vi "Stop Work.vi"(6 "Controller name":string, 8 "error in (no error)":errorcluster, 9 "Reply":bool=TRUE, 10 "Reply to":refnum<class "Stop Response Msg.lvclass">, 11 "Measure Object in":refnum<class "Channel Scanner.lvclass">) -> (0 "error out":errorcluster, 3 "Measure Object out":refnum<class "Channel Scanner.lvclass">)   [LabVIEW 2021, in "Channel Scanner.lvclass"]
uses:
  Channel Scanner.lvclass
  C:/Program Files/National Instruments/LabVIEW 2021/vi.lib/ActorFramework/Actor/Actor.lvclass
  Controllers/Process Controller Messages/Stop Response Msg/Stop Response Msg.lvclass
  <vilib>/ActorFramework/Actor/Actor.lvclass/Actor.ctl
  <vilib>/ActorFramework/Message Enqueuer/Message Enqueuer.lvclass/Message Enqueuer.ctl
  Publish-Subscribe/Interfaces/Publisher Messages/Unsubscribe Msg/Unsubscribe Msg.lvclass/Unsubscribe Msg.ctl
  <vilib>/ActorFramework/Message Enqueuer/Init from Existing Queue.vi
  <vilib>/ActorFramework/Message Enqueuer/Enqueue.vi
  Publish-Subscribe/Interfaces/Publisher Messages/Unsubscribe Msg/Unsubscribe Msg.lvclass
  C:/Program Files/National Instruments/LabVIEW 2021/vi.lib/ActorFramework/Message/Message.lvclass
  <vilib>/ActorFramework/Message Priority Queue/Priority Enqueue.vi
  Instrument Actor/Instrument Actor.lvclass
  <vilib>/ActorFramework/Message Enqueuer/Message Enqueuer.lvclass
  <vilib>/ActorFramework/Actor/Actor.lvclass
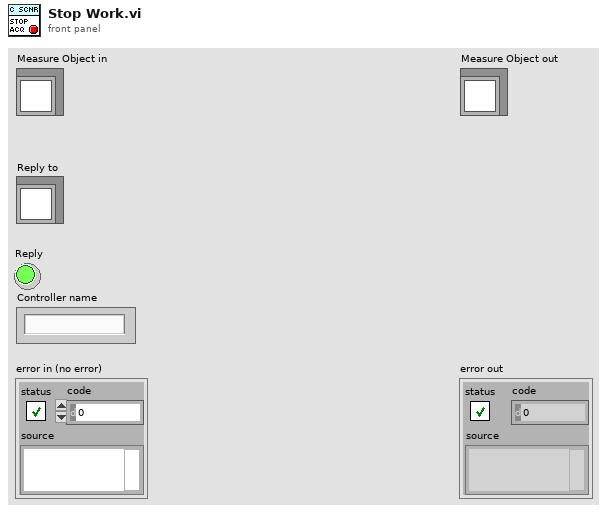
[diagram p1: front panel]
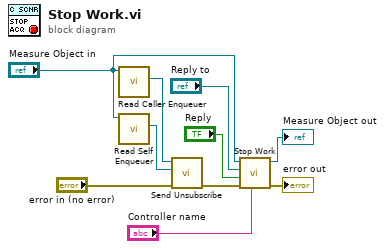
[diagram p0: block diagram]
diagram:
  n1 = call <vilib>:"Read Caller Enqueuer.vi"("Actor"="Measure Object in") -> ("Caller Enqueuer"=w4:refnum<class "Message Enqueuer.lvclass">)  [unwired: 10 in]
  n2 = call <vilib>:"Read Self Enqueuer.vi"("Actor"="Measure Object in") -> ("Self Enqueuer"=w5:refnum<class "Message Enqueuer.lvclass">)  [unwired: 10 in]
  n3 = call "Send Unsubscribe.vi"("error in (no error)"="error in (no error)", "Subscriber Enq"=w5, "Message Enqueuer"=w4) -> ("error out"=w2:errorcluster)  [unwired: 7 in, 1 out]
  n4 = call-parent "Stop Work.vi"("Controller name"="Controller name", "error in (no error)"=w2, "Reply"="Reply", "Reply to"="Reply to", "Measure Object in"="Measure Object in") -> ("error out"=→"error out":errorcluster, "Measure Object out"=→"Measure Object out":refnum<class "Channel Scanner.lvclass">)  [unwired: 5 in]
